vi "Neocera21 Set Heater.vi"(8 "error in (no error)":errorcluster, 10 "Set T":T1, 11 "VISA Resource Name":refnum<visa-resource-name>) -> (0 "error out":errorcluster, 3 "VISA Resource Name Out":refnum<visa-resource-name>)   [LabVIEW 2015]
uses:
  Neocera Heater Ranges.ctl
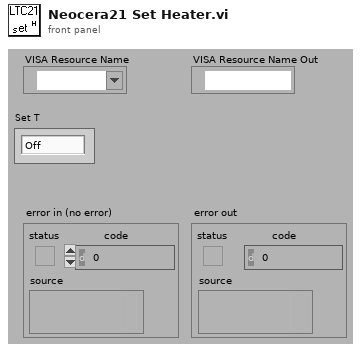
[diagram p1: front panel]
types:
  T1 = typedef "Neocera Heater Ranges.ctl" = enum16{"Off", "0.05W", "0.5W", "5W", "50W"}
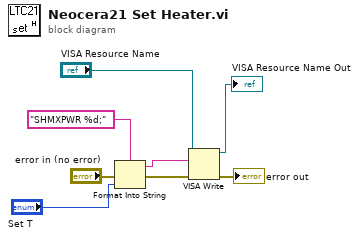
[diagram p0: block diagram]
diagram:
  n1 = Format Into String(format string="SHMXPWR %d;" ("data string"), error in="error in (no error)", "Set T") -> (resulting string=w1:string, error out=w2:errorcluster)  [unwired: 1 in]
  n2 = VISA Write(VISA resource name="VISA Resource Name", write buffer=w1, error in (no error)=w2) -> (VISA resource name out=→"VISA Resource Name Out":refnum<visa-resource-name>, error out=→"error out":errorcluster)  [unwired: 1 out]
